vi "Reset (Set).vi"(6 "ISOBUS address":T3=-1 caption="ISOBUS address (-1)", 8 "error in":errorcluster, 11 "Mercury Reference In":T4) -> (0 "error out":errorcluster, 2 "Response":T2, 3 "Mercury Reference Out":T4, 4 "Valid?":T1)   [LabVIEW 2014, in "Mercury iXX.lvlib" / "System.lvlib"]
doc: "Reset the instrument.\n\nThis will cause the instrument to reboot and the user will need to reselect the remote mode on the instrument."
uses:
  System.lvlib
  Controls/Mercury Reference.ctl
  Controls/Comms Transport Layer.ctl
  Private/Controls/Query Dynamic Reference.ctl
  Controls/ISOBus Address.ctl
  Controls/Response String.ctl
  Controls/Is Valid LED.ctl
  Mercury iXX.lvlib
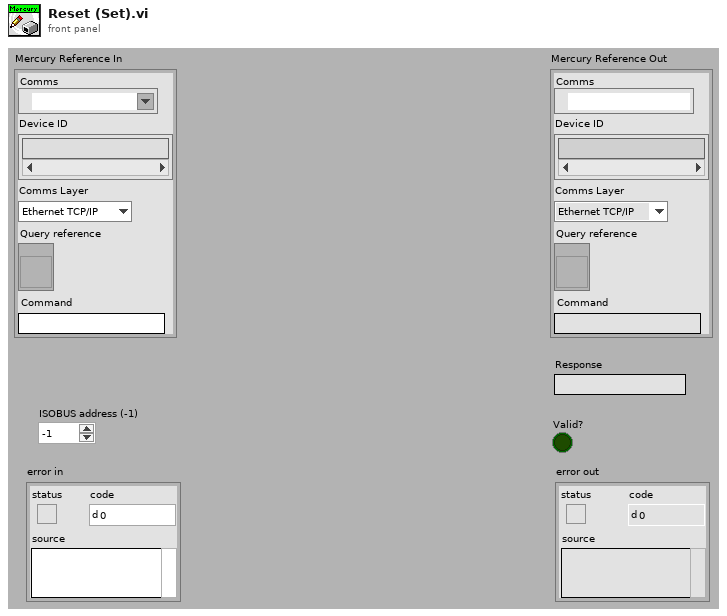
[diagram p1: front panel]
types:
  T1 = typedef "Mercury iXX.lvlib/Is Valid LED.ctl" = bool
  T2 = typedef "Mercury iXX.lvlib/Response String.ctl" = string
  T3 = typedef "Mercury iXX.lvlib/ISOBus Address.ctl" = i32
  T4 = typedef "Mercury iXX.lvlib/Mercury Reference.ctl" = cluster{"Comms":refnum<visa-resource-name>, "Device ID":string[], "Comms Layer":T5, "Command":string, "Query reference":T6}
  T5 = typedef "Mercury iXX.lvlib/Comms Transport Layer.ctl" = enum16{"Ethernet TCP/IP", "USB", "ISOBus - RS-232", "GPIB"}
  T6 = typedef "Mercury iXX.lvlib/Query Dynamic Reference.ctl" = refnum<vi>
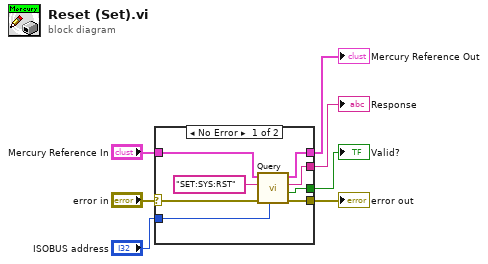
[diagram p0: block diagram]
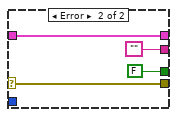
[diagram p2: hidden frame]
diagram:
  n1 = case shown="No Error" "error in" {
    selector: "error in" -> [w12 w18]
    tunnel: "Mercury Reference In" -> [w15 w19]
    tunnel: [w13 w19] -> w6
    tunnel: [w14 w18] -> w5
    tunnel: "ISOBUS address" -> [w10 _]
    tunnel: [w9 ""] -> w2
    tunnel: [w8 FALSE ("Valid?")] -> w1
    frame No Error {
      n2 = call "Query.vi"("ISOBUS address"=w10, "error in"=w12, "Command"="SET:SYS:RST", "Mercury Reference In"=w15) -> ("error out"=w14:errorcluster, "Valid?"=w8:bool, "Data"=w9:string, "Mercury Reference Out"=w13:T4)  [unwired: 1 in, 3 out]
    }
    frame Error {
    }
  }
  "Mercury Reference Out" <- w6
  "error out" <- w5
  "Response" <- w2
  "Valid?" <- w1
